vi "Add Alarm Folder_Alarm Folder.vi"(8 "error in (no error)":errorcluster, 9 "Alarm Folder":T1, 11 "Alarms Ref":refnum<k24>) -> (0 "error out":errorcluster, 3 "Alarms Ref out":refnum<k24>)   [LabVIEW 2019, in "Simple SysDef API.lvlib"]
uses:
  <userlib>/SimpleSysDef/Simple SysDef API.lvlib
  NationalInstruments.VeriStand.SystemDefinitionAPI
  <userlib>/SimpleSysDef/_SubVIs/Add Alarm Folder_Settings.ctl
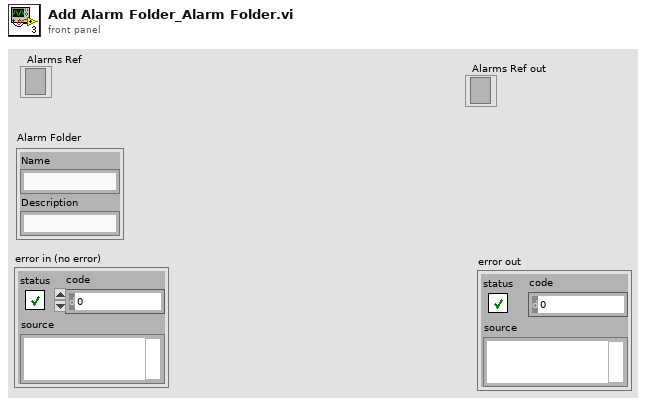
[diagram p1: front panel]
types:
  T1 = typedef "Simple SysDef API.lvlib/Add Alarm Folder_Settings.ctl" = cluster{"Name":string, "Description":string}
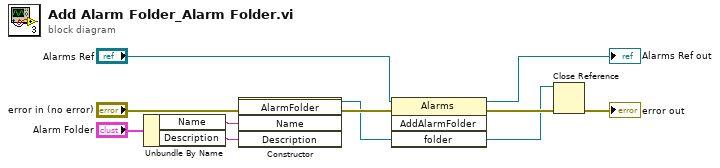
[diagram p0: block diagram]
diagram:
  n1 = Unbundle By Name("Alarm Folder") -> ("Name"=w1:string, "Description"=w2:string)
  n2 = constructor class="AlarmFolder"(error in="error in (no error)", "Name"=w1, "Description"=w2) -> (reference out=w7:refnum<k24>, error out=w9:errorcluster)  [unwired: 2 in, 3 out]
  n3 = invoke class="Alarms" method="AddAlarmFolder"(reference="Alarms Ref", error in=w9, "folder"=w7) -> (reference out=→"Alarms Ref out":refnum<k24>, error out=w8:errorcluster)  [unwired: 1 in, 2 out]
  n4 = Close Reference(reference=w7, error in (no error)=w8) -> (error out=→"error out":errorcluster)
